vi "AlazarSetTriggerOperation.vi"(0 "Handle":u64, 1 "Trigger Operation":u32(ring) items=["J", "K", "J OR K", "J AND K", "J XOR K", "J AND NOT K", "NOT J AND K"], 5 "error in (no error)":errorcluster, 6 "Trigger Engine 1":u32(ring) items=["J", "K"], 7 "Trigger Engine 2":u32(ring)=1 items=["J", "K"], 8 "Source 1":u32(ring) items=["A", "B", "External", "Disable", "C", "D"], 9 "Source 2":u32(ring)=3 items=["A", "B", "External", "Disable", "C", "D"], 10 "Slope 1":u32(ring)=1 items=["Positive"=1, "Negative"=2], 11 "Slope 2":u32(ring)=1 items=["Positive"=1, "Negative"=2], 12 "Level 1":u32, 13 "Level 2":u32) -> (14 "Handle":u64, 18 "Return Code":u32, 19 "error out":errorcluster)   [LabVIEW 2018]
doc: "Configure the trigger system."
uses:
  ATSApi.dll
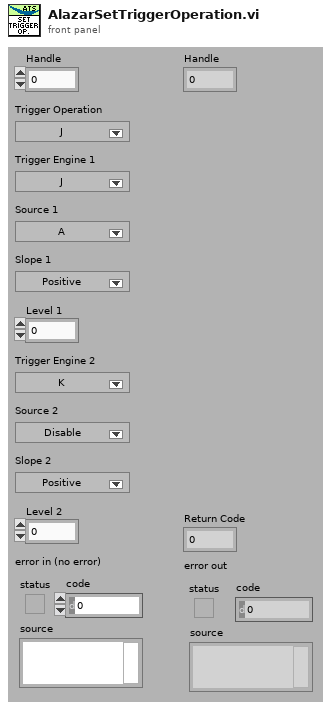
[diagram p1: front panel]
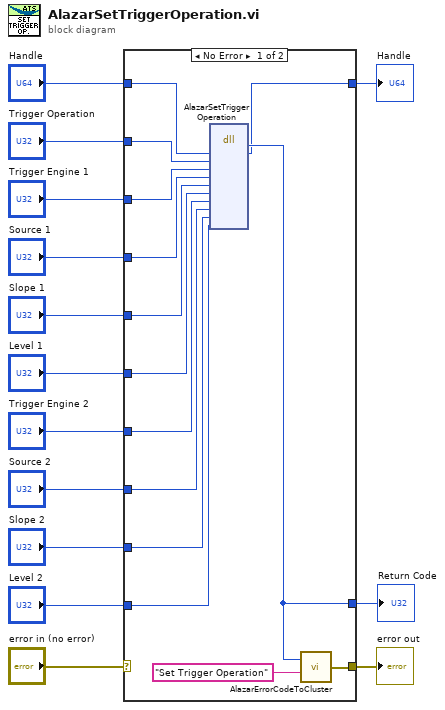
[diagram p0: block diagram]
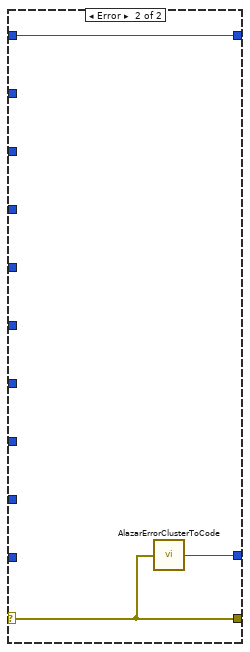
[diagram p2: hidden frame]
diagram:
  n1 = case shown="No Error" "error in (no error)" {
    selector: "error in (no error)" -> [_ w31]
    tunnel: [w25 w31] -> w13
    tunnel: [w27 w30] -> w12
    tunnel: "Handle" -> [w28 w29]
    tunnel: [w24 w29] -> w10
    tunnel: "Trigger Operation" -> [w23 _]
    tunnel: "Trigger Engine 1" -> [w22 _]
    tunnel: "Source 1" -> [w21 _]
    tunnel: "Slope 1" -> [w20 _]
    tunnel: "Level 1" -> [w19 _]
    tunnel: "Trigger Engine 2" -> [w18 _]
    tunnel: "Source 2" -> [w17 _]
    tunnel: "Slope 2" -> [w16 _]
    tunnel: "Level 2" -> [w15 _]
    frame No Error {
      n2 = dll-call lib="ATSApi.dll" fn="AlazarSetTriggerOperation"("handle"=w28, "triggerOperation"=w23, "triggerEngine1"=w22, "source1"=w21, "slope1"=w20, "level1"=w19, "triggerEngine2"=w18, "source2"=w17, "slope2"=w16, "level2"=w15) -> ("return type"=w27:u32, "handle"=w24:u64)  [unwired: 12 in, 2 out]
      n3 = call "AlazarErrorCodeToCluster.vi"("Message"="Set Trigger Operation", "Error Code"=w27) -> ("error out"=w25:errorcluster)
    }
    frame Error {
      n4 = call "AlazarErrorClusterToCode.vi"("error in (no error)"=w31) -> ("Error Code"=w30:u32)
    }
  }
  "Handle" <- w10
  "error out" <- w13
  "Return Code" <- w12
